vi "GetAnalogDataType.vi"(1 "Task ID":u32) -> (0 "return type":i32)   [LabVIEW 2015]
uses:
  Windows/System32/AdvLvDaq.dll
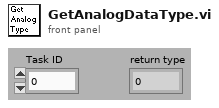
[diagram p1: front panel]
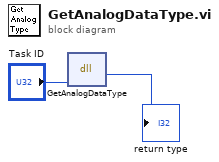
[diagram p0: block diagram]
diagram:
  n1 = dll-call lib="C:/Windows/System32/AdvLvDaq.dll" fn="GetAnalogDataType"("taskId"="Task ID") -> ("return type"=→"return type":i32)  [unwired: 4 in, 2 out]
